vi "rotate.vi"(8 "degrees to  rotate":dbl, 9 "right(T)/left(F)":bool, 10 "power":u16=75, 11 "NXT 2":T1={"Hardware"="NXT", "Flattened String"=""}) -> (3 "NXT":T1={"Hardware"="NXT", "Flattened String"=""})   [LabVIEW 2012]
uses:
  <vilib>/NXT/Subs/LVHSConnector.ctl
  <vilib>/NXT/Subs/MotorOutput.ctl
  <vilib>/NXT/Dual Mode Library/Waits/Wait_Num(msec).vi
  <vilib>/NXT/Dual Mode Library/Motors/MotorBrake.vi
  <vilib>/NXT/Dual Mode Library/Motors/MotorOn.vi
  <vilib>/NXT/Dual Mode Library/Motors/MotorReverse.vi
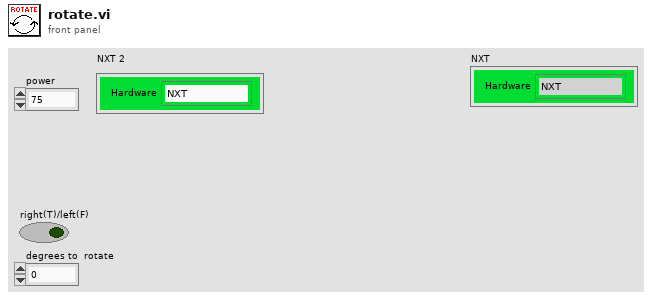
[diagram p1: front panel]
types:
  T1 = typedef "LVHSConnector.ctl" = cluster{"Hardware":string, "Flattened String":string}
  T2 = typedef "MotorOutput.ctl" = u8
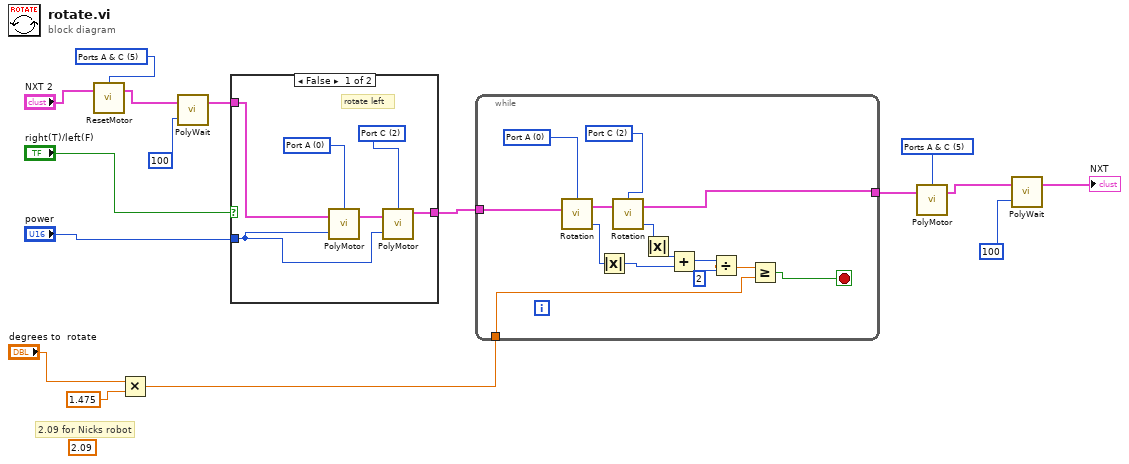
[diagram p0: block diagram]
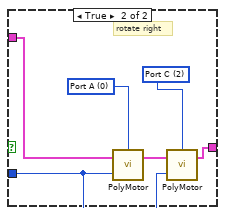
[diagram p2: hidden frame]
diagram:
  w4 = T2 5 items=["Port A"=0, "Port B"=1, "Port C"=2, "Ports A & B"=4, "Ports A & C"=5, "Ports B & C"=6, "All Ports"=3] ("Port (All Ports)")
  (unwired) 2.09 ("Max Value")
  w12 = T2 5 items=["Port A"=0, "Port B"=1, "Port C"=2, "Ports A & B"=4, "Ports A & C"=5, "Ports B & C"=6, "All Ports"=3] ("Port (All Ports)")
  # "2.09 for Nicks robot"
  n1 = call <vilib>:"ResetMotor.vi"("NXT"="NXT 2", "Port (All Ports)"=w4) -> ("NXT"=w2:T1)  [unwired: 2 in]
  n2 = Multiply(x="degrees to  rotate", y=1.475 ("Max Value")) -> (x*y=w11:dbl)
  n3 = call-poly <vilib>:"PolyWait.vi"("Time (100 msec)"=i16 100 ("y"), "NXT"=w2) -> ("NXT"=w1:T1)  [unwired: 2 in]
  n4 = case shown="False" "right(T)/left(F)" {
    tunnel: "power" -> [w18 w24]
    tunnel: w1 -> [w17 w23]
    tunnel: [w19 w25] -> w15
    frame False {
      w22 = T2 2 items=["Port A"=0, "Port B"=1, "Port C"=2, "Ports A & B"=4, "Ports A & C"=5, "Ports B & C"=6, "as"=3] ("Output Port (All Ports)")
      w20 = T2 0 items=["Port A"=0, "Port B"=1, "Port C"=2, "Ports A & B"=4, "Ports A & C"=5, "Ports B & C"=6, "as"=3] ("Output Port (All Ports)")
      # "rotate left"
      n5 = call-poly <vilib>:"PolyMotor.vi"("Power (75)"=w18, "NXT"=w17, "Output Port (All Ports)"=w20) -> ("NXT"=w21:T1)  [unwired: 1 in]
      n6 = call-poly <vilib>:"PolyMotor.vi"("Power (75)"=w18, "NXT"=w21, "Output Port (All Ports)"=w22) -> ("NXT"=w19:T1)  [unwired: 1 in]
    }
    frame True {
      w28 = T2 2 items=["Port A"=0, "Port B"=1, "Port C"=2, "Ports A & B"=4, "Ports A & C"=5, "Ports B & C"=6, "as"=3] ("Output Port (All Ports)")
      w26 = T2 0 items=["Port A"=0, "Port B"=1, "Port C"=2, "Ports A & B"=4, "Ports A & C"=5, "Ports B & C"=6, "as"=3] ("Output Port (All Ports)")
      # "rotate right"
      n7 = call-poly <vilib>:"PolyMotor.vi"("Power (75)"=w24, "NXT"=w23, "Output Port (All Ports)"=w26) -> ("NXT"=w27:T1)  [unwired: 1 in]
      n8 = call-poly <vilib>:"PolyMotor.vi"("Power (75)"=w24, "NXT"=w27, "Output Port (All Ports)"=w28) -> ("NXT"=w25:T1)  [unwired: 1 in]
    }
  }
  n9 = while {
    tunnel: w15 -> [w42]
    tunnel: w11 -> [w32]
    tunnel: [w29] -> w13
    stop <- w30 stop-if-true
    w39 = T2 2 items=["Port A"=0, "Port B"=1, "Port C"=2, "Ports A & B"=4, "Ports A & C"=5, "Ports B & C"=6, "as"=3] ("Output Port (All Ports)")
    w40 = T2 0 items=["Port A"=0, "Port B"=1, "Port C"=2, "Ports A & B"=4, "Ports A & C"=5, "Ports B & C"=6, "as"=3] ("Output Port (All Ports)")
    n10 = call <vilib>:"Rotation.vi"("NXT"=w42, "Port (Port A)"=w40) -> ("Angle of Rotation"=w38:i32, "NXT"=w41:T1)  [unwired: 1 in]
    n11 = Absolute Value(x=w38) -> (abs(x)=w36:i32)
    n12 = call <vilib>:"Rotation.vi"("NXT"=w41, "Port (Port A)"=w39) -> ("Angle of Rotation"=w37:i32, "NXT"=w29:T1)  [unwired: 1 in]
    n13 = Absolute Value(x=w37) -> (abs(x)=w35:i32)
    n14 = Add(x=w35, y=w36) -> (x+y=w34:i32)
    n15 = Divide(x=w34, y=2) -> (x/y=w31:dbl)
    n16 = Greater Or Equal?(x=w31, y=w32) -> (x >= y?=w30:bool)
  }
  n17 = call-poly <vilib>:"PolyMotor.vi"("NXT"=w13, "Port (All Ports)"=w12) -> ("NXT"=w7:T1)  [unwired: 2 in]
  n18 = call-poly <vilib>:"PolyWait.vi"("Time (100 msec)"=i16 100 ("y"), "NXT"=w7) -> ("NXT"=→"NXT":T1)  [unwired: 2 in]
